vi "Save_Cluster_to_Text_File.vi"() -> ()   [LabVIEW 2025]
panel:
  out "Results History":string
  in  "stop":bool
  in  "Read":bool
  in  "Save":bool
  in  "Test Cluster":T1
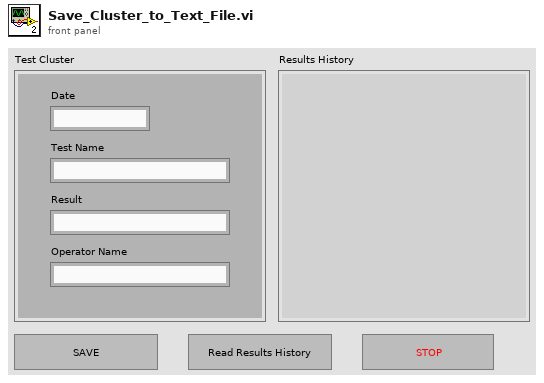
[diagram p1: front panel]
types:
  T1 = cluster{"Date":string, "Test Name":string, "Result":string, "Operator Name":string}
  T2 = enum16{"open", "replace", "create", "open or create", "replace or create", "replace or create with confirmation"}
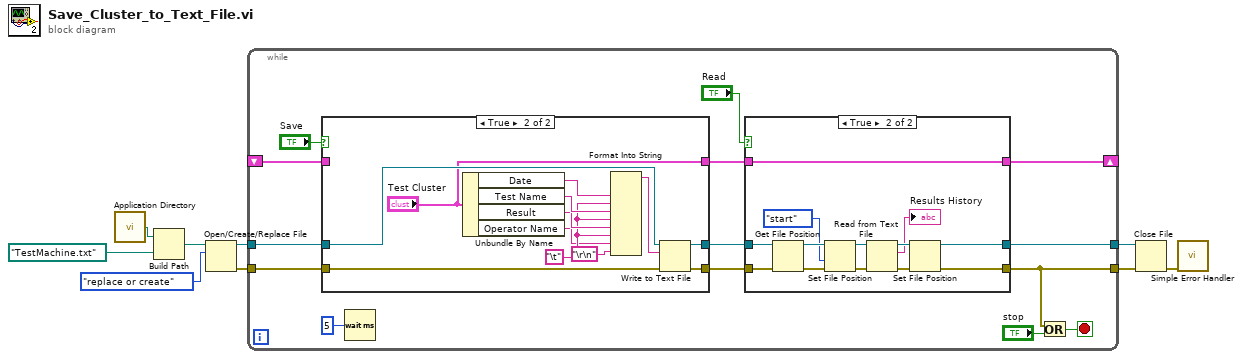
[diagram p0: block diagram]
diagram:
  n1 = call <vilib>:"Application Directory.vi"() -> ("Application Directory"=w9:path)
  n2 = Build Path(base path=w9, name or relative path=path "TestMachine.txt") -> (appended path=w7:path)
  n3 = Open/Create/Replace File(file path (use dialog)=w7, operation (0:open)=T2."replace or create") -> (refnum out=w5:refnum<file>, error out=w4:errorcluster)  [unwired: 4 in, 1 out]
  n4 = while {
    tunnel: w5 -> [w22]
    tunnel: w4 -> [w21]
    tunnel: [w14] -> w3
    tunnel: [w16] -> w2
    shift-right: [w11] -> _
    shift-left: _ -> [w10]
    stop <- w13 stop-if-true
    n5 = case shown="True" "Save" {
      tunnel: w22 -> [w41 w48]
      tunnel: w21 -> [w40 w47]
      tunnel: [w40 w45] -> w18
      tunnel: [w41 w44] -> w17
      tunnel: [w42 "Test Cluster"] -> w12
      tunnel: w10 -> [w42 _]
      frame False {
      }
      frame True {
        w51 = "\t"
        n6 = Unbundle By Name("Test Cluster") -> ("Date"=w54:string, "Test Name"=w53:string, "Result"=w52:string, "Operator Name"=w50:string)
        n7 = Format Into String(w54, w51, w53, w51, w52, w51, w50, "\r\n") -> (resulting string=w46:string)  [unwired: 3 in, 1 out]
        n8 = Write to Text File(file (use dialog)=w48, text=w46, error in=w47) -> (refnum out=w44:refnum<file>, error out=w45:errorcluster)  [unwired: 1 in, 1 out]
      }
    }
    n9 = Wait (ms)(milliseconds to wait=u32 5) -> ()  [unwired: 1 out]
    n10 = case shown="True" "Read" {
      tunnel: w18 -> [w24 w39]
      tunnel: [w24 w35] -> w14
      tunnel: w17 -> [w25 w34]
      tunnel: [w25 w30] -> w16
      tunnel: w12 -> [w26 w27]
      tunnel: [w26 w27] -> w11
      frame False {
      }
      frame True {
        n11 = Get File Position(4:w39, 7:w34) -> (0:w38:errorcluster, 3:w33:refnum<file>)  [unwired: 1 out]
        n12 = Set File Position(refnum=w33, from (0:start)=enum16{"start", "end", "current"}."start", error in=w38) -> (refnum out=w32:refnum<file>, error out=w37:errorcluster)  [unwired: 1 in]
        n13 = Read from Text File(file (use dialog)=w32, error in=w37) -> (refnum out=w31:refnum<file>, text=→"Results History":string, error out=w36:errorcluster)  [unwired: 2 in, 1 out]
        n14 = Set File Position(refnum=w31, error in=w36) -> (refnum out=w30:refnum<file>, error out=w35:errorcluster)  [unwired: 2 in]
      }
    }
    n15 = Or(x=w14, y="stop") -> (x .or. y?=w13:bool)
  }
  n16 = Close File(refnum=w2, error in=w3) -> (error out=w1:errorcluster)  [unwired: 1 out]
  n17 = call <vilib>:"Simple Error Handler.vi"("error in (no error)"=w1) -> ()  [unwired: 4 in, 5 out]
